vi "Random Number Within Range - I32__ogtk.vi"(0 "High":i32=1, 1 "Low":i32) -> (4 "Random Number":i32)   [LabVIEW 2020]
doc: "Generates a <b>Random Number</b> between <b>High</b> and <b>Low</b> inputs. Prechecks data to ensure that <b>High</b> is greater than <b>Low</b>."
panel:
  # "Please visit http://www.OpenG.org to learn about the\nOpen Source LabVIEW software movement.\n\nNOTICE -- YOU MUST LEAVE THIS NOTICE IN PLACE.  PER THE TERMS OF THE LICENSE BELOW, YOU MAY SUBLICENSE THIS SOFTWARE \nIN ANY WAY THAT DOES NOT CONFLICT WITH THIS LICENSE.\n\n### BSD License (http://www.opensource.org/licenses/bsd-license.php) Begin ###\n \nCopyright (c) 2002-2011, Jim Kring <jim@jimkring.com>\nCopyright (c) 2011, Jonathon Green <jg@jgcode.net>\n\nAll rights reserved.\n\nRedistribution and use in source and binary forms, with or without modification, are permitted provided that the following conditions are met:\n\n    * Redistributions of source code must retain the above copyright notice, this list of conditions and the following disclaimer.\n    * Redistributions in binary form must reproduce the above copyright notice, this list of conditions and the following disclaimer in the \n       documentation and/or other materials provided with the distribution.\n    * Neither the name of SciWare, James Kring, Inc., nor the names of its contributors may be used to endorse or promote products derived \n       from this software without specific prior written permission.\n\nTHIS SOFTWARE IS PROVIDED BY THE COPYRIGHT HOLDERS AND CONTRIBUTORS \"AS IS\" AND ANY EXPRESS OR IMPLIED WARRANTIES, \nINCLUDING, BUT NOT LIMITED TO, THE IMPLIED WARRANTIES OF MERCHANTABILITY AND FITNESS FOR A PARTICULAR PURPOSE ARE \nDISCLAIMED. IN NO EVENT SHALL THE COPYRIGHT OWNER OR CONTRIBUTORS BE LIABLE FOR ANY DIRECT, INDIRECT, INCIDENTAL,\n SPECIAL, EXEMPLARY, OR CONSEQUENTIAL DAMAGES (INCLUDING, BUT NOT LIMITED TO, PROCUREMENT OF SUBSTITUTE GOODS OR \nSERVICES; LOSS OF USE, DATA, OR PROFITS; OR BUSINESS INTERRUPTION) HOWEVER CAUSED AND ON ANY THEORY OF LIABILITY, \nWHETHER IN CONTRACT, STRICT LIABILITY, OR TORT (INCLUDING NEGLIGENCE OR OTHERWISE) ARISING IN ANY WAY OUT OF THE USE \nOF THIS SOFTWARE, EVEN IF ADVISED OF THE POSSIBILITY OF SUCH DAMAGE.\n\n### BSD License End ###"
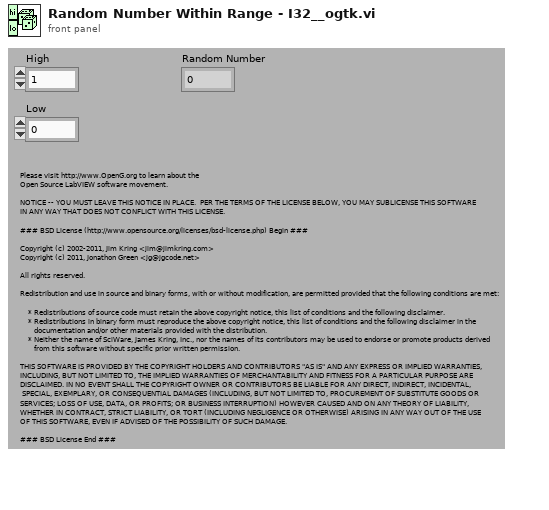
[diagram p1: front panel]
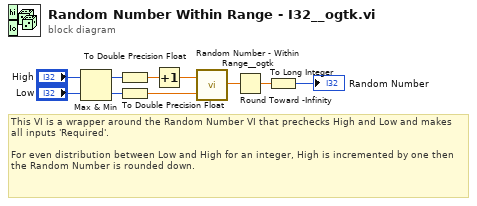
[diagram p0: block diagram]
diagram:
  # "This VI is a wrapper around the Random Number VI that prechecks High and Low and makes all inputs 'Required'.\n\nFor even distribution between Low and High for an integer, High is incremented by one then the Random Number is rounded down."
  n1 = Max & Min(x="High", y="Low") -> (max(x,y)=w7:i32, min(x,y)=w5:i32)
  n2 = To Double Precision Float(number=w7) -> (double precision float=w6:dbl)
  n3 = To Double Precision Float(number=w5) -> (double precision float=w3:dbl)
  n4 = Increment(x=w6) -> (x+1=w4:dbl)
  n5 = call "Random Number - Within Range__ogtk.vi"("High (1.00)"=w4, "Low (0.00)"=w3) -> ("Random Number"=w2:dbl)  [unwired: 3 in]
  n6 = Round Toward -Infinity(1:w2) -> (0:w8:dbl)
  n7 = To Long Integer(number=w8) -> (32bit integer=→"Random Number":i32)
